vi "Add Server Connection.vi"(8 "error in (no error)":errorcluster, 10 "Connection":variant, 11 "RemoteControl.STM in":refnum<class "RemoteControl.STM.lvclass">) -> (0 "error out":errorcluster, 3 "RemoteControl.STM out":refnum<class "RemoteControl.STM.lvclass">)   [LabVIEW 2016, in "RemoteControl.STM.lvclass"]
uses:
  RemoteControl.STM.lvclass
  RemoteControl.STM.lvclass/RemoteControl.STM.ctl
  <vilib>/NI/STM/TCP/Get Connection Reference (TCP).vi
  <vilib>/NI/STM/TCP/Write Meta Data (TCP Ref).vi
  <vilib>/NI/STM/TCP/Write Meta Data (TCP Clst).vi
  RemoteControl/RemoteControl.lvclass
  <vilib>/NI/STM/NI STM.lvlib
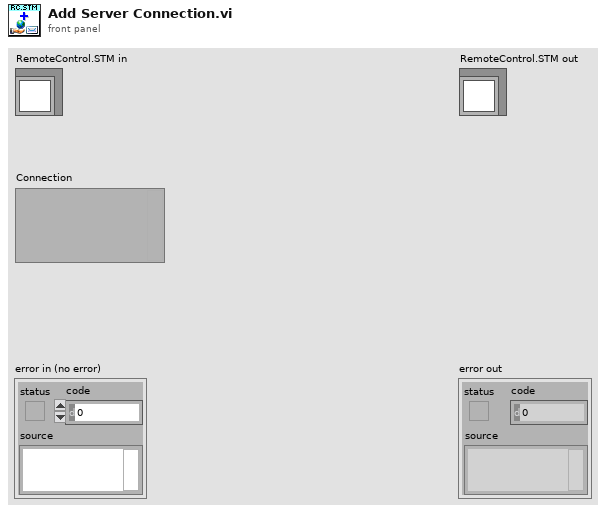
[diagram p1: front panel]
types:
  T1 = typedef "NI STM.lvlib/MetaDataElement.ctl" = string
  T2 = typedef "NI STM.lvlib/TCP Connection Info.ctl" = cluster{"connection ID":refnum<k5>, "meta data":T1[]}
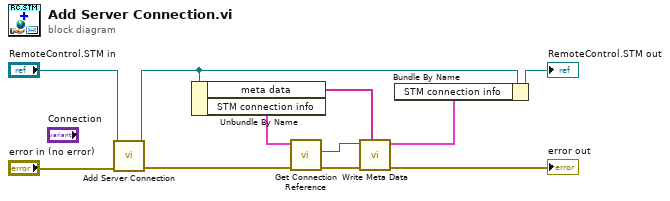
[diagram p0: block diagram]
diagram:
  n1 = call-parent "Add Server Connection.vi"("error in (no error)"="error in (no error)", "RemoteControl in"="RemoteControl.STM in") -> ("error out"=w6:errorcluster, "RemoteControl out"=w4:refnum<class "RemoteControl.STM.lvclass">)  [unwired: 8 in]
  n2 = Unbundle By Name(w4) -> ("meta data"=w8:T1[], "STM connection info"=w10:T2)
  n3 = call-poly <vilib>:"Get Connection Reference.vi"("error in"=w6, "connection info in"=w10) -> ("error out"=w7:errorcluster, "connection ID out"=w9:refnum<k5>)  [unwired: 7 in, 1 out]
  n4 = call-poly <vilib>:"Write Meta Data.vi"("meta data"=w8, "error in"=w7, "connection ID"=w9) -> ("error out"=→"error out":errorcluster, "connection info out"=w1:T2)  [unwired: 7 in]
  n5 = Bundle By Name(cluster=w4, "STM connection info"=w1) -> (→"RemoteControl.STM out":refnum<class "RemoteControl.STM.lvclass">)
